vi "SetTDSegLen.vi"(8 "error in":errorcluster, 11 "SegLen":u8) -> (0 "error out":errorcluster)   [LabVIEW 2012]
uses:
  bin/OVA32.dll
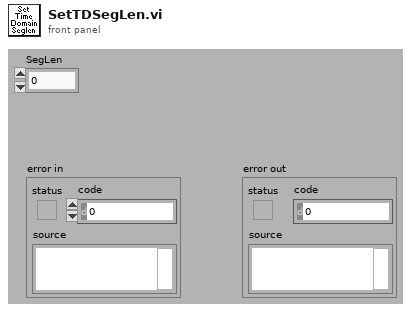
[diagram p1: front panel]
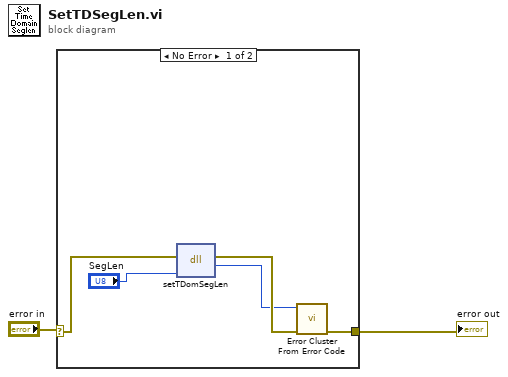
[diagram p0: block diagram]
diagram:
  n1 = case shown="No Error" "error in" {
    selector: "error in" -> [w6 w8]
    tunnel: [w7 w8] -> w1
    frame No Error {
      n2 = dll-call lib="C:/_src/OVA5000_DSP_falcon/Software/LabVIEW/OVA/SDK/OVA_5000_SDK_v5.14.3/bin/OVA32.dll" fn="setTDomSegLen"(error in=w6, "arg1"="SegLen") -> (error out=w5:errorcluster, "return type"=w4:i32)  [unwired: 3 in, 1 out]
      n3 = call <vilib>:"Error Cluster From Error Code.vi"("error in (no error)"=w5, "error code (0)"=w4) -> ("error out"=w7:errorcluster)  [unwired: 7 in]
    }
    frame Error {
    }
  }
  "error out" <- w1
